vi "Stage Message Loop.vi"(8 "error in (no error)":errorcluster, 11 "Message Queues":T2) -> (0 "error out":errorcluster)   [LabVIEW 2017, in "Stage.lvlib"]
uses:
  Stage.lvlib
  Vibratome/Message Queues.ctl
  Support VIs/Message Queue/Message.ctl
  Controller States.ctl
  Drivers/ASI/Public/Utility/Axis Name.ctl
  Set Point States.ctl
  <vilib>/Utility/error.llb/Error Cluster From Error Code.vi
  Support VIs/Message Queue/Enqueue Message (Single).vi
  Support VIs/Message Queue/Enqueue Message (Multiple).vi
  <vilib>/ErrorRing/Error Ring.xnode
  Support VIs/Message Queue/Message Queue.lvlib
  Drivers/ASI/ASI TG-1000.lvlib
  Vibratome/Vibratome.lvlib
panel:
  out "Controller State":T1
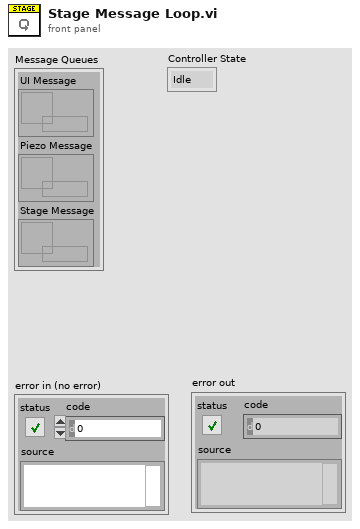
[diagram p1: front panel]
types:
  T1 = typedef "Stage.lvlib/Controller States.ctl" = enum16{"Idle", "Jog", "Busy"}
  T2 = typedef "Vibratome.lvlib/Message Queues.ctl" = cluster{"UI Message":refnum<queue>, "Piezo Message":refnum<queue>, "Stage Message":refnum<queue>}
  T3 = typedef "Drivers.lvlib/ASI TG-1000.lvlib/Axis Name.ctl" = enum8{"undefined", "A", "B", "C", "D", "E", "F", "G", "H", "I", "J", "K", "L", "M", "N", "O", "P", "Q", "R", "S", "T", "U", "V", "W", "X", "Y", "Z"}
  T4 = cluster{"start":dbl, "end":dbl, "cut speed":dbl, "max speed":dbl, "thickness":dbl, "active axis":T3, "jog step":dbl, "pos?":bool, "x step":dbl}
  T5 = typedef "Stage.lvlib/Set Point States.ctl" = enum16{"Unset", "Setting", "Ready"}
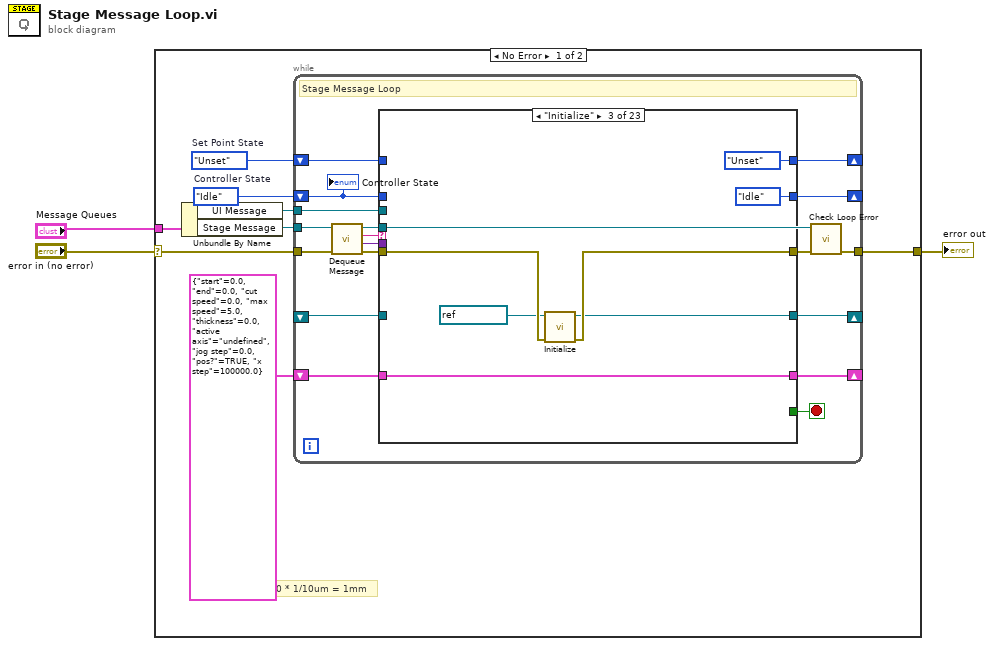
[diagram p0: block diagram]
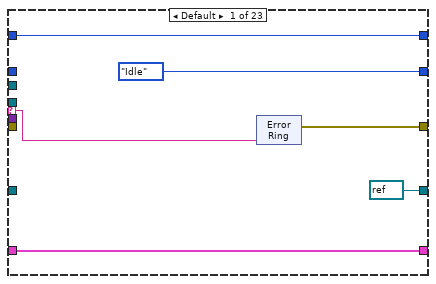
[diagram p2: hidden frame]
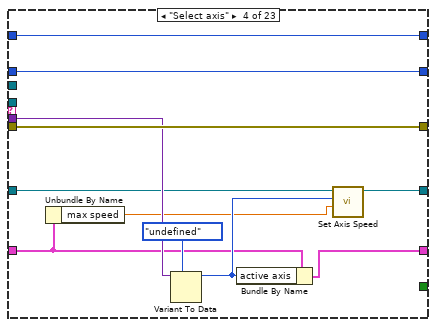
[diagram p4: hidden frame]
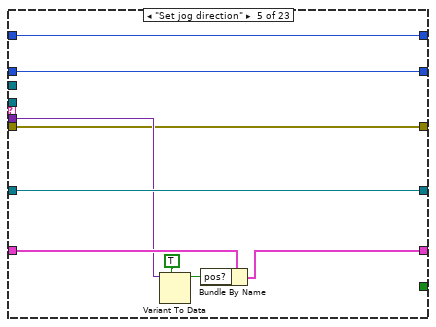
[diagram p5: hidden frame]
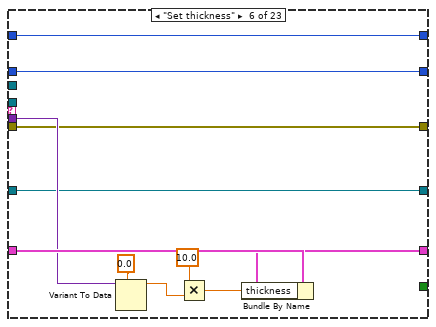
[diagram p6: hidden frame]
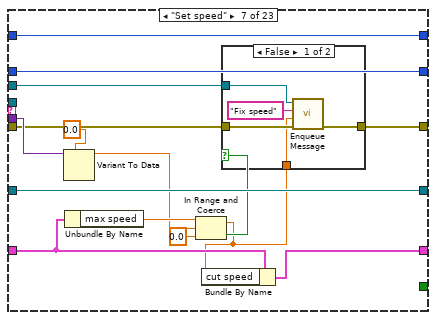
[diagram p7: hidden frame]
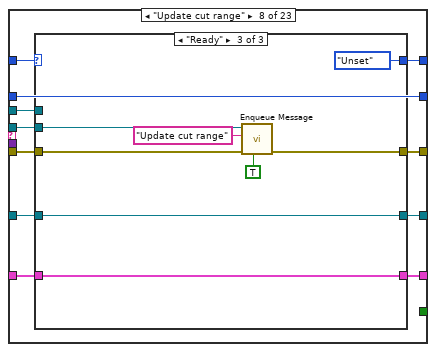
[diagram p9: hidden frame]
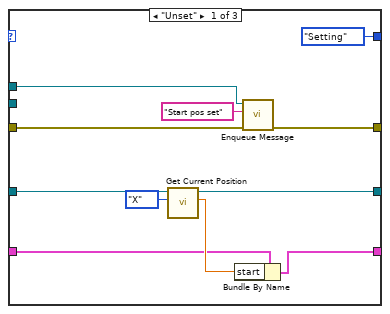
[diagram p10: hidden frame]
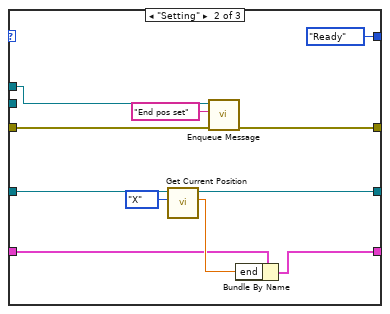
[diagram p11: hidden frame]
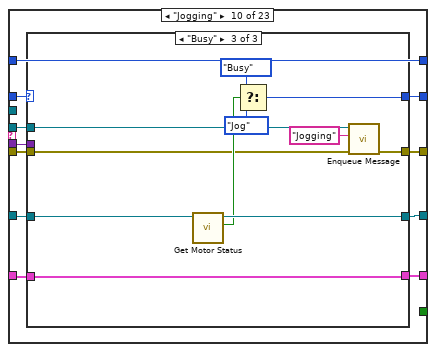
[diagram p13: hidden frame]
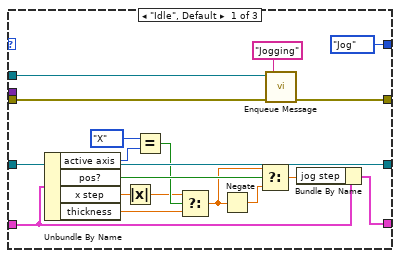
[diagram p14: hidden frame]
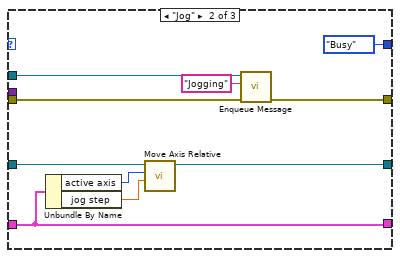
[diagram p15: hidden frame]
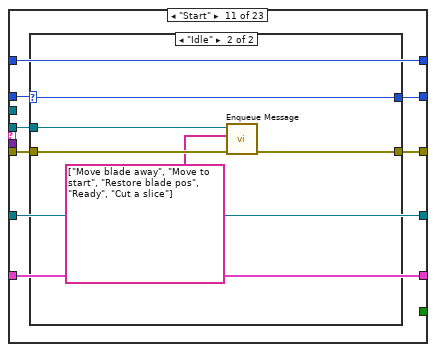
[diagram p16: hidden frame]
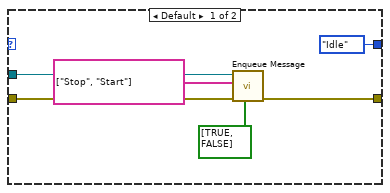
[diagram p17: hidden frame]
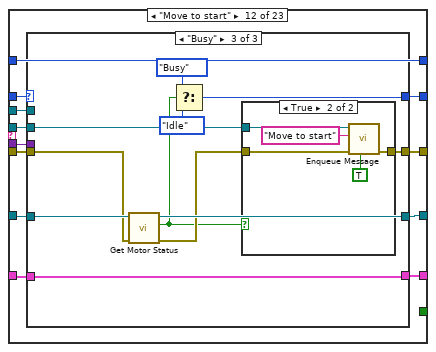
[diagram p18: hidden frame]
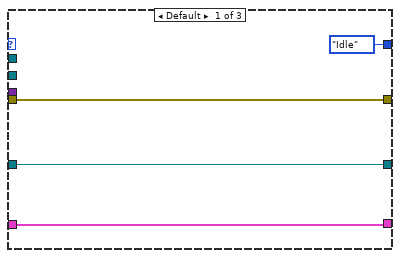
[diagram p19: hidden frame]
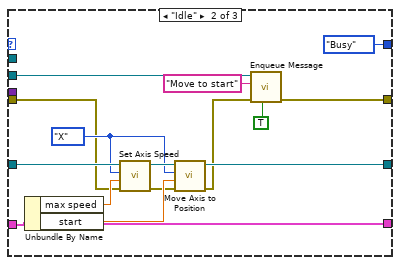
[diagram p20: hidden frame]
diagram:
  n1 = case shown="No Error" "error in (no error)" {
    selector: "error in (no error)" -> [w10 w531]
    tunnel: "Message Queues" -> [w11 _]
    tunnel: [w8 w531] -> w1
    frame No Error {
      w4 = Controller_States."Idle"  # Controller State
      w5 = Set_Point_States."Unset"  # Set Point State
      # "1000 0 * 1/10um = 1mm"
      n2 = Unbundle By Name(w11) -> ("UI Message"=w6:refnum<queue>, "Stage Message"=w9:refnum<queue>)
      n3 = while {
        tunnel: w10 -> [w29]
        tunnel: w9 -> [w23]
        tunnel: [w22] -> w8
        shift-right: [w20] -> _
        shift-left: _ -> [w19]
        shift-right: [w17] -> _
        shift-left: T4 {"start"=0.0, "end"=0.0, "cut speed"=0.0, "max speed"=5.0, "thickness"=0.0, "active axis"=enum."undefined", "jog step"=0.0, "pos?"=TRUE, "x step"=100000.0} -> [w18]
        shift-right: [w15] -> _
        shift-left: w4 -> [w16]
        tunnel: w6 -> [w14]
        shift-right: [w12] -> _
        shift-left: w5 -> [w13]
        stop <- w24 stop-if-true
        # "Stage Message Loop"
        n4 = call "Dequeue Message.vi"("error in (no error)"=w29, "Message Queue in"=w23) -> ("error out"=w27:errorcluster, "Data"=w21:variant, "State"=w28:string, "Message Queue out"=w26:refnum<queue>)  [unwired: 6 in]
        n5 = case shown="\"Initialize\"" w28 {
          selector: w28 -> [w34 _ _ _ _ _ _ _ _ _ _ _ _ _ _ _ _ _ _ _ _ _ _]
          tunnel: w26 -> [_ _ _ _ _ _ _ w109 _ w154 w209 w224 _ w284 w295 w347 w358 w406 w455 w506 _ _ _]
          tunnel: w27 -> [_ w47 w54 w64 w70 w80 w89 w110 w152 w157 w208 w227 w275 w283 w298 w346 w361 w409 w458 w510 w517 w522 w528]
          tunnel: [w35 w47 w52 w64 w70 w80 w90 w108 w152 w156 w207 w226 w274 w282 w297 w345 w360 w408 w457 w511 w517 w522 w527] -> w25
          tunnel: [_ _ _ _ _ _ _ _ _ _ _ _ _ _ _ _ _ _ _ _ _ _ TRUE] -> w24
          tunnel: w21 -> [_ _ _ w62 w71 w84 w96 _ _ w158 _ w228 _ _ w299 _ w362 w410 w459 _ _ _ _]
          tunnel: [refnum<visa-resource-name> refnum ("VISA resource name out") w46 w51 w59 w74 w81 w99 w115 w151 w160 w206 w230 w271 w281 w301 w344 w364 w412 w461 w509 w516 w521 refnum<visa-resource-name> refnum ("VISA out")] -> w20
          tunnel: w19 -> [_ w46 _ w60 w74 w81 w99 w116 w151 w159 w206 w229 w271 w281 w300 w344 w363 w411 w460 w508 w516 w521 w529]
          tunnel: w18 -> [w32 w45 w48 w57 w73 w85 w93 w113 w150 w162 w205 w232 w270 w280 w303 w343 w366 w414 w463 w507 w515 w520 w525]
          tunnel: [w32 w45 w48 w63 w67 w78 w92 w114 w150 w161 w205 w231 w270 w280 w302 w343 w365 w413 w462 w507 w515 w520 w525] -> w17
          tunnel: w16 -> [_ w44 _ w65 w69 w79 w100 w111 w149 w163 w204 w233 w276 w279 w304 w342 w367 w415 w464 _ w514 _ _]
          tunnel: [Controller_States."Idle" w44 Controller_States."Idle" w65 w69 w79 w100 w111 w149 w155 w203 w225 w276 w278 w296 w341 w359 w407 w456 Controller_States."Idle" w514 Controller_States."Idle" Controller_States."Idle"] -> w15
          tunnel: w14 -> [_ _ _ _ _ _ w88 w107 _ _ _ w222 w273 _ w293 _ w356 w404 w453 w504 _ _ _]
          tunnel: w13 -> [w30 w43 _ w55 w66 w77 w86 w117 w148 w153 w210 w223 w277 w285 w294 w348 w357 w405 w454 w505 w513 w518 w523]
          tunnel: [w30 w43 Set_Point_States."Unset" ("Set Point State") w55 w66 w77 w86 w112 w148 w153 w210 w223 w277 w285 w294 w348 w357 w405 w454 w505 w513 w518 w523] -> w12
          frame Default {
            n6 = xnode "Error Ring"("parameter 0"=w34) -> ("error out"=w35:errorcluster)
          }
          frame "--- SETUP ---" {
          }
          frame "Initialize" {
            n7 = call "Initialize.vi"("error in (no error)"=w54, "VISA resource name"=refnum<visa-resource-name> "COM13") -> ("error out"=w52:errorcluster, "VISA resource name out"=w51:refnum<visa-resource-name>)  [unwired: 8 in]
          }
          frame "Select axis" {
            n8 = Unbundle By Name(w57) -> ("max speed"=w56:dbl)
            n9 = Variant To Data(type=Axis_Name."undefined" ("active axis"), Variant=w62) -> (data=w58:T3)  [unwired: 1 in, 1 out]
            n10 = Bundle By Name(cluster=w57, "active axis"=w58) -> (w63:T4)
            n11 = call "Set Axis Speed.vi"("Speed (mm/s)"=w56, "Axis"=w58, "VISA resource name"=w60) -> ("VISA out"=w59:refnum<visa-resource-name>)  [unwired: 7 in, 1 out]
          }
          frame "Set jog direction" {
            n12 = Variant To Data(type=TRUE, Variant=w71) -> (data=w68:bool)  [unwired: 1 in, 1 out]
            n13 = Bundle By Name(cluster=w73, "pos?"=w68) -> (w67:T4)
          }
          frame "Set thickness" {
            n14 = Variant To Data(type=0.0, Variant=w84) -> (data=w82:dbl)  [unwired: 1 in, 1 out]
            n15 = Multiply(x=10.0, y=w82) -> (x*y=w76:dbl)
            n16 = Bundle By Name(cluster=w85, "thickness"=w76) -> (w78:T4)
          }
          frame "Set speed" {
            n17 = Variant To Data(type=0.0, Variant=w96) -> (data=w95:dbl)  [unwired: 1 in, 1 out]
            n18 = Unbundle By Name(w93) -> ("max speed"=w98:dbl)
            n19 = In Range and Coerce(upper limit=w98, x=w95, lower limit=0.0) -> (coerced(x)=w87:dbl, In Range?=w91:bool)
            n20 = Bundle By Name(cluster=w93, "cut speed"=w87) -> (w92:T4)
            n21 = case shown="False" w91 {
              tunnel: [w104 w106] -> w90
              tunnel: w89 -> [w105 w106]
              tunnel: w88 -> [w103 _]
              tunnel: w87 -> [w101 _]
              frame False {
                n22 = call-poly "Enqueue Message.vi"("error in (no error)"=w105, "Data"=w101, "State"="Fix speed", "Message Queue in"=w103) -> ("error out"=w104:errorcluster)  [unwired: 6 in, 1 out]
              }
              frame True {
              }
            }
          }
          frame "Update cut range" {
            n23 = case shown="\"Ready\"" w117 {
              tunnel: w116 -> [w128 w139 w145]
              tunnel: [w127 w138 w145] -> w115
              tunnel: [w123 w134 w146] -> w114
              tunnel: w113 -> [w124 w135 w146]
              tunnel: [Set_Point_States."Setting" ("Set Point State") Set_Point_States."Ready" ("Set Point State") Set_Point_States."Unset" ("Set Point State")] -> w112
              tunnel: w110 -> [w121 w131 w144]
              tunnel: w109 -> [_ _ w143]
              tunnel: [w120 w130 w140] -> w108
              tunnel: w107 -> [w119 w132 _]
              frame "Unset" {
                n24 = call "Get Current Position.vi"("Axis"=Axis_Name."X", "VISA in"=w128) -> ("position [internal units]"=w125:dbl, "VISA out"=w127:refnum<visa-resource-name>)  [unwired: 7 in, 1 out]
                n25 = Bundle By Name(cluster=w124, "start"=w125) -> (w123:T4)
                n26 = call-poly "Enqueue Message.vi"("error in (no error)"=w121, "State"="Start pos set", "Message Queue in"=w119) -> ("error out"=w120:errorcluster)  [unwired: 7 in, 1 out]
              }
              frame "Setting" {
                n27 = call "Get Current Position.vi"("Axis"=Axis_Name."X", "VISA in"=w139) -> ("position [internal units]"=w136:dbl, "VISA out"=w138:refnum<visa-resource-name>)  [unwired: 7 in, 1 out]
                n28 = call-poly "Enqueue Message.vi"("error in (no error)"=w131, "State"="End pos set", "Message Queue in"=w132) -> ("error out"=w130:errorcluster)  [unwired: 7 in, 1 out]
                n29 = Bundle By Name(cluster=w135, "end"=w136) -> (w134:T4)
              }
              frame "Ready" {
                n30 = call-poly "Enqueue Message.vi"("High Priority?"=TRUE, "error in (no error)"=w144, "State"="Update cut range", "Message Queue in"=w143) -> ("error out"=w140:errorcluster)  [unwired: 6 in, 1 out]
              }
            }
          }
          frame "--- OPS ---" {
          }
          frame "Jogging" {
            n31 = case shown="\"Busy\"" w163 {
              tunnel: w162 -> [w175 w188 w202]
              tunnel: [w178 w188 w202] -> w161
              tunnel: [w177 w182 w200] -> w160
              tunnel: w159 -> [w177 w184 w201]
              tunnel: w158 -> [_ _ _]
              tunnel: w157 -> [w173 w189 w195]
              tunnel: [w172 w190 w194] -> w156
              tunnel: [Controller_States."Jog" Controller_States."Busy" w197] -> w155
              tunnel: w154 -> [w174 w187 w193]
              frame "Idle", Default {
                n32 = Unbundle By Name(w175) -> ("active axis"=w169:T3, "pos?"=w170:bool, "x step"=w181:dbl, "thickness"=w165:dbl)
                n33 = Absolute Value(x=w181) -> (abs(x)=w166:dbl)
                n34 = Equal?(x=Axis_Name."X", y=w169) -> (x = y?=w167:bool)
                n35 = Select(t=w166, s=w167, f=w165) -> (s? t:f=w164:dbl)
                n36 = Negate(x=w164) -> (-x=w180:dbl)
                n37 = Select(t=w164, s=w170, f=w180) -> (s? t:f=w179:dbl)
                n38 = call-poly "Enqueue Message.vi"("error in (no error)"=w173, "State"="Jogging", "Message Queue in"=w174) -> ("error out"=w172:errorcluster)  [unwired: 7 in, 1 out]
                n39 = Bundle By Name(cluster=w175, "jog step"=w179) -> (w178:T4)
              }
              frame "Jog" {
                n40 = Unbundle By Name(w188) -> ("active axis"=w185:T3, "jog step"=w183:dbl)
                n41 = call "Move Axis Relative.vi"("Relative Position [internal units]"=w183, "Axis"=w185, "VISA in"=w184) -> ("VISA out"=w182:refnum<visa-resource-name>)  [unwired: 6 in, 1 out]
                n42 = call-poly "Enqueue Message.vi"("error in (no error)"=w189, "State"="Jogging", "Message Queue in"=w187) -> ("error out"=w190:errorcluster)  [unwired: 7 in, 1 out]
              }
              frame "Busy" {
                n43 = call "Get Motor Status.vi"("VISA in"=w201) -> ("Motors Busy?"=w199:bool, "VISA out"=w200:refnum<visa-resource-name>)  [unwired: 7 in, 1 out]
                n44 = Select(t=Controller_States."Busy", s=w199, f=Controller_States."Jog") -> (s? t:f=w197:T1)
                n45 = call-poly "Enqueue Message.vi"("error in (no error)"=w195, "State"="Jogging", "Message Queue in"=w193) -> ("error out"=w194:errorcluster)  [unwired: 7 in, 1 out]
              }
            }
          }
          frame "Start" {
            n46 = case shown="\"Idle\"" w204 {
              selector: w204 -> [_ w217]
              tunnel: w209 -> [w215 w221]
              tunnel: w208 -> [w214 w220]
              tunnel: [w213 w219] -> w207
              tunnel: [Controller_States."Idle" ("Controller State") w217] -> w203
              frame Default {
                n47 = call-poly "Enqueue Message.vi"("Priority Message?"=bool[] [TRUE, FALSE], "error in (no error)"=w214, "States"=string[] ["Stop", "Start"], "Message Queue in"=w215) -> ("error out"=w213:errorcluster)  [unwired: 6 in, 1 out]
              }
              frame "Idle" {
                n48 = call-poly "Enqueue Message.vi"("error in (no error)"=w220, "States"=string[] ["Move blade away", "Move to start", "Restore blade pos", "Ready", "Cut a slice"], "Message Queue in"=w221) -> ("error out"=w219:errorcluster)  [unwired: 7 in, 1 out]
              }
            }
          }
          frame "Move to start" {
            n49 = case shown="\"Busy\"" w233 {
              tunnel: w232 -> [w234 w251 w263]
              tunnel: [w234 w251 w263] -> w231
              tunnel: [w235 w248 w261] -> w230
              tunnel: w229 -> [w235 w252 w262]
              tunnel: w228 -> [_ _ _]
              tunnel: w227 -> [w236 w239 w255]
              tunnel: [w236 w242 w257] -> w226
              tunnel: [Controller_States."Idle" ("f") Controller_States."Busy" ("f") w259] -> w225
              tunnel: w224 -> [_ w244 w256]
              tunnel: w222 -> [_ _ _]
              frame Default {
              }
              frame "Idle" {
                w247 = Axis_Name."X" ("Axis")
                n50 = Unbundle By Name(w251) -> ("max speed"=w250:dbl, "start"=w246:dbl)
                n51 = call "Set Axis Speed.vi"("error in (no error)"=w239, "Speed (mm/s)"=w250, "Axis"=w247, "VISA resource name"=w252) -> ("error out"=w240:errorcluster, "VISA out"=w249:refnum<visa-resource-name>)  [unwired: 6 in]
                n52 = call "Move Axis to Position.vi"("error in (no error)"=w240, "Position [internal units]"=w246, "Axis"=w247, "VISA in"=w249) -> ("error out"=w238:errorcluster, "VISA out"=w248:refnum<visa-resource-name>)  [unwired: 5 in]
                n53 = call-poly "Enqueue Message.vi"("High Priority?"=TRUE, "error in (no error)"=w238, "State"="Move to start", "Message Queue in"=w244) -> ("error out"=w242:errorcluster)  [unwired: 6 in, 1 out]
              }
              frame "Busy" {
                n54 = call "Get Motor Status.vi"("error in (no error)"=w255, "VISA in"=w262) -> ("error out"=w254:errorcluster, "Motors Busy?"=w253:bool, "VISA out"=w261:refnum<visa-resource-name>)  [unwired: 6 in]
                n55 = Select(t=Controller_States."Busy", s=w253, f=Controller_States."Idle") -> (s? t:f=w259:T1)
                n56 = case shown="True" w253 {
                  tunnel: [w264 w269] -> w257
                  tunnel: w256 -> [_ w268]
                  tunnel: w254 -> [w264 w266]
                  frame False {
                  }
                  frame True {
                    n57 = call-poly "Enqueue Message.vi"("High Priority?"=TRUE, "error in (no error)"=w266, "State"="Move to start", "Message Queue in"=w268) -> ("error out"=w269:errorcluster)  [unwired: 6 in, 1 out]
                  }
                }
              }
            }
          }
          frame "Ready" {
            n58 = call-poly "Enqueue Message.vi"("error in (no error)"=w275, "State"="Started", "Message Queue in"=w273) -> ("error out"=w274:errorcluster)  [unwired: 7 in, 1 out]
          }
          frame "Cut a slice" {
            n59 = case shown="\"Idle\"" w279 {
              selector: w279 -> [_ w288]
              tunnel: w284 -> [_ w292]
              tunnel: w283 -> [w286 w291]
              tunnel: [w286 w290] -> w282
              tunnel: [Controller_States."Idle" ("Controller State") w288] -> w278
              frame Default {
              }
              frame "Idle" {
                n60 = call-poly "Enqueue Message.vi"("error in (no error)"=w291, "States"=string[] ["Move to end", "Prepare for next slice", "Cut a slice"], "Message Queue in"=w292) -> ("error out"=w290:errorcluster)  [unwired: 7 in, 1 out]
              }
            }
          }
          frame "Move to end" {
            n61 = case shown="\"Busy\"" w304 {
              tunnel: w303 -> [w305 w322 w334]
              tunnel: [w305 w322 w334] -> w302
              tunnel: [w306 w319 w332] -> w301
              tunnel: w300 -> [w306 w323 w333]
              tunnel: w299 -> [_ _ _]
              tunnel: w298 -> [w307 w310 w326]
              tunnel: [w307 w313 w328] -> w297
              tunnel: [Controller_States."Idle" ("f") Controller_States."Busy" ("f") w330] -> w296
              tunnel: w295 -> [_ w315 w327]
              tunnel: w293 -> [_ _ _]
              frame Default {
              }
              frame "Idle" {
                w318 = Axis_Name."X" ("Axis")
                n62 = Unbundle By Name(w322) -> ("cut speed"=w321:dbl, "end"=w317:dbl)
                n63 = call "Set Axis Speed.vi"("error in (no error)"=w310, "Speed (mm/s)"=w321, "Axis"=w318, "VISA resource name"=w323) -> ("error out"=w311:errorcluster, "VISA out"=w320:refnum<visa-resource-name>)  [unwired: 6 in]
                n64 = call "Move Axis to Position.vi"("error in (no error)"=w311, "Position [internal units]"=w317, "Axis"=w318, "VISA in"=w320) -> ("error out"=w309:errorcluster, "VISA out"=w319:refnum<visa-resource-name>)  [unwired: 5 in]
                n65 = call-poly "Enqueue Message.vi"("High Priority?"=TRUE, "error in (no error)"=w309, "State"="Move to end", "Message Queue in"=w315) -> ("error out"=w313:errorcluster)  [unwired: 6 in, 1 out]
              }
              frame "Busy" {
                n66 = call "Get Motor Status.vi"("error in (no error)"=w326, "VISA in"=w333) -> ("error out"=w325:errorcluster, "Motors Busy?"=w324:bool, "VISA out"=w332:refnum<visa-resource-name>)  [unwired: 6 in]
                n67 = Select(t=Controller_States."Busy", s=w324, f=Controller_States."Idle") -> (s? t:f=w330:T1)
                n68 = case shown="True" w324 {
                  tunnel: [w335 w340] -> w328
                  tunnel: w327 -> [_ w339]
                  tunnel: w325 -> [w335 w337]
                  frame False {
                  }
                  frame True {
                    n69 = call-poly "Enqueue Message.vi"("High Priority?"=TRUE, "error in (no error)"=w337, "State"="Move to end", "Message Queue in"=w339) -> ("error out"=w340:errorcluster)  [unwired: 6 in, 1 out]
                  }
                }
              }
            }
          }
          frame "Prepare for next slice" {
            n70 = case shown="\"Idle\"" w342 {
              selector: w342 -> [_ w351]
              tunnel: w347 -> [_ w355]
              tunnel: w346 -> [w349 w354]
              tunnel: [w349 w353] -> w345
              tunnel: [Controller_States."Idle" ("Controller State") w351] -> w341
              frame Default {
              }
              frame "Idle" {
                n71 = call-poly "Enqueue Message.vi"("error in (no error)"=w354, "States"=string[] ["Move blade away", "Move to start", "Restore blade pos", "Move up one slice"], "Message Queue in"=w355) -> ("error out"=w353:errorcluster)  [unwired: 7 in, 1 out]
              }
            }
          }
          frame "Move blade away" {
            n72 = case shown="\"Idle\"" w367 {
              tunnel: w366 -> [w368 w385 w397]
              tunnel: [w368 w385 w397] -> w365
              tunnel: [w369 w375 w395] -> w364
              tunnel: w363 -> [w369 w386 w396]
              tunnel: w362 -> [_ _ _]
              tunnel: w361 -> [w370 w378 w389]
              tunnel: [w370 w380 w391] -> w360
              tunnel: [Controller_States."Idle" ("f") Controller_States."Busy" ("f") w393] -> w359
              tunnel: w358 -> [_ w382 w390]
              tunnel: w356 -> [_ _ _]
              frame Default {
              }
              frame "Idle" {
                w373 = Axis_Name."F" ("Axis")
                n73 = Unbundle By Name(w385) -> ("max speed"=w384:dbl, "thickness"=w372:dbl)
                n74 = call "Set Axis Speed.vi"("error in (no error)"=w378, "Speed (mm/s)"=w384, "Axis"=w373, "VISA resource name"=w386) -> ("error out"=w377:errorcluster, "VISA out"=w376:refnum<visa-resource-name>)  [unwired: 6 in]
                n75 = call "Move Axis Relative.vi"("error in (no error)"=w377, "Relative Position [internal units]"=w372, "Axis"=w373, "VISA in"=w376) -> ("error out"=w374:errorcluster, "VISA out"=w375:refnum<visa-resource-name>)  [unwired: 5 in]
                n76 = call-poly "Enqueue Message.vi"("High Priority?"=TRUE, "error in (no error)"=w374, "State"="Move blade away", "Message Queue in"=w382) -> ("error out"=w380:errorcluster)  [unwired: 6 in, 1 out]
              }
              frame "Busy" {
                n77 = call "Get Motor Status.vi"("error in (no error)"=w389, "VISA in"=w396) -> ("error out"=w388:errorcluster, "Motors Busy?"=w387:bool, "VISA out"=w395:refnum<visa-resource-name>)  [unwired: 6 in]
                n78 = Select(t=Controller_States."Busy", s=w387, f=Controller_States."Idle") -> (s? t:f=w393:T1)
                n79 = case shown="False" w387 {
                  tunnel: [w398 w403] -> w391
                  tunnel: w390 -> [_ w402]
                  tunnel: w388 -> [w398 w400]
                  frame False {
                  }
                  frame True {
                    n80 = call-poly "Enqueue Message.vi"("High Priority?"=TRUE, "error in (no error)"=w400, "State"="Move blade away", "Message Queue in"=w402) -> ("error out"=w403:errorcluster)  [unwired: 6 in, 1 out]
                  }
                }
              }
            }
          }
          frame "Restore blade pos" {
            n81 = case shown="\"Idle\"" w415 {
              tunnel: w414 -> [w416 w434 w446]
              tunnel: [w416 w434 w446] -> w413
              tunnel: [w417 w424 w444] -> w412
              tunnel: w411 -> [w417 w435 w445]
              tunnel: w410 -> [_ _ _]
              tunnel: w409 -> [w418 w427 w438]
              tunnel: [w418 w429 w440] -> w408
              tunnel: [Controller_States."Idle" ("f") Controller_States."Busy" ("f") w442] -> w407
              tunnel: w406 -> [_ w431 w439]
              tunnel: w404 -> [_ _ _]
              frame Default {
              }
              frame "Idle" {
                w422 = Axis_Name."F" ("Axis")
                n82 = Unbundle By Name(w434) -> ("max speed"=w433:dbl, "thickness"=w421:dbl)
                n83 = Negate(x=w421) -> (-x=w420:dbl)
                n84 = call "Set Axis Speed.vi"("error in (no error)"=w427, "Speed (mm/s)"=w433, "Axis"=w422, "VISA resource name"=w435) -> ("error out"=w426:errorcluster, "VISA out"=w425:refnum<visa-resource-name>)  [unwired: 6 in]
                n85 = call "Move Axis Relative.vi"("error in (no error)"=w426, "Relative Position [internal units]"=w420, "Axis"=w422, "VISA in"=w425) -> ("error out"=w423:errorcluster, "VISA out"=w424:refnum<visa-resource-name>)  [unwired: 5 in]
                n86 = call-poly "Enqueue Message.vi"("High Priority?"=TRUE, "error in (no error)"=w423, "State"="Restore blade pos", "Message Queue in"=w431) -> ("error out"=w429:errorcluster)  [unwired: 6 in, 1 out]
              }
              frame "Busy" {
                n87 = call "Get Motor Status.vi"("error in (no error)"=w438, "VISA in"=w445) -> ("error out"=w437:errorcluster, "Motors Busy?"=w436:bool, "VISA out"=w444:refnum<visa-resource-name>)  [unwired: 6 in]
                n88 = Select(t=Controller_States."Busy", s=w436, f=Controller_States."Idle") -> (s? t:f=w442:T1)
                n89 = case shown="False" w436 {
                  tunnel: [w447 w452] -> w440
                  tunnel: w439 -> [_ w451]
                  tunnel: w437 -> [w447 w449]
                  frame False {
                  }
                  frame True {
                    n90 = call-poly "Enqueue Message.vi"("High Priority?"=TRUE, "error in (no error)"=w449, "State"="Restore blade pos", "Message Queue in"=w451) -> ("error out"=w452:errorcluster)  [unwired: 6 in, 1 out]
                  }
                }
              }
            }
          }
          frame "Move up one slice" {
            n91 = case shown="\"Busy\"" w464 {
              tunnel: w463 -> [w465 w482 w494]
              tunnel: [w465 w482 w494] -> w462
              tunnel: [w466 w472 w492] -> w461
              tunnel: w460 -> [w466 w483 w493]
              tunnel: w459 -> [_ _ _]
              tunnel: w458 -> [w467 w475 w486]
              tunnel: [w467 w477 w488] -> w457
              tunnel: [Controller_States."Idle" ("f") Controller_States."Busy" ("f") w490] -> w456
              tunnel: w455 -> [_ w479 w487]
              tunnel: w453 -> [_ _ _]
              frame Default {
              }
              frame "Idle" {
                w470 = Axis_Name."Z" ("Axis")
                n92 = Unbundle By Name(w482) -> ("max speed"=w481:dbl, "thickness"=w469:dbl)
                n93 = call "Set Axis Speed.vi"("error in (no error)"=w475, "Speed (mm/s)"=w481, "Axis"=w470, "VISA resource name"=w483) -> ("error out"=w474:errorcluster, "VISA out"=w473:refnum<visa-resource-name>)  [unwired: 6 in]
                n94 = call "Move Axis Relative.vi"("error in (no error)"=w474, "Relative Position [internal units]"=w469, "Axis"=w470, "VISA in"=w473) -> ("error out"=w471:errorcluster, "VISA out"=w472:refnum<visa-resource-name>)  [unwired: 5 in]
                n95 = call-poly "Enqueue Message.vi"("High Priority?"=TRUE, "error in (no error)"=w471, "State"="Move up one slice", "Message Queue in"=w479) -> ("error out"=w477:errorcluster)  [unwired: 6 in, 1 out]
              }
              frame "Busy" {
                n96 = call "Get Motor Status.vi"("error in (no error)"=w486, "VISA in"=w493) -> ("error out"=w485:errorcluster, "Motors Busy?"=w484:bool, "VISA out"=w492:refnum<visa-resource-name>)  [unwired: 6 in]
                n97 = Select(t=Controller_States."Busy", s=w484, f=Controller_States."Idle") -> (s? t:f=w490:T1)
                n98 = case shown="True" w484 {
                  tunnel: [w495 w500] -> w488
                  tunnel: w487 -> [_ w499]
                  tunnel: w485 -> [w495 w497]
                  frame False {
                  }
                  frame True {
                    n99 = call-poly "Enqueue Message.vi"("High Priority?"=TRUE, "error in (no error)"=w497, "State"="Move up one slice", "Message Queue in"=w499) -> ("error out"=w500:errorcluster)  [unwired: 6 in, 1 out]
                  }
                }
              }
            }
          }
          frame "Stop" {
            n100 = Flush Queue(queue=w506, error in (no error)=w510) -> (error out=w503:errorcluster)  [unwired: 2 out]
            n101 = call "Halt all Commands.vi"("error in (no error)"=w503, "VISA in"=w508) -> ("error out"=w502:errorcluster, "VISA out"=w509:refnum<visa-resource-name>)  [unwired: 7 in]
            n102 = call-poly "Enqueue Message.vi"("error in (no error)"=w502, "State"="Stopped", "Message Queue in"=w504) -> ("error out"=w511:errorcluster)  [unwired: 7 in, 1 out]
          }
          frame "--- MISC ---" {
          }
          frame "Error" {
          }
          frame "Exit" {
            n103 = call "Close.vi"("error in (no error)"=w528, "VISA resource name"=w529) -> ("error out"=w527:errorcluster)  [unwired: 9 in]
          }
        }
        n104 = call "Check Loop Error.vi"("error in (no error)"=w25, "Message Queue in"=w26) -> ("error out"=w22:errorcluster)  [unwired: 7 in, 2 out]
        "Controller State" <- w16
      }
    }
    frame Error {
    }
  }
  "error out" <- w1
